vi "teste_command_final.vi"() -> ()   [LabVIEW 2025]
uses:
  <vilib>/Plasmionique/MB Master/MB_Master_Serial/MB_Master_Serial.lvclass
  C:/Program Files/National Instruments/LabVIEW 2025/vi.lib/Plasmionique/MB Master/MB_Master/MB_Master.lvclass
panel:
  out "error out":errorcluster
  in  "habilitar":u16=256
  in  "velocidade":u16
  in  "Serial Config":T1={"baud rate (bps)"=9600, "stop bits"=10, "parity"=2, "flow control"=0, "timeout"=2000, "retries"=3} {"stop bits" items=["1.0"=10, "1.5"=15, "2.0"=20]; "flow control" items=["None", "XON/XOFF", "RTS/CTS", "XON/XOFF & RTS/CTS", "DTR/DSR", "XON/XOFF & DTR/DSR"]; "parity" items=["None", "Odd", "Even", "Mark", "Space"]}
  in  "VISA Resource":refnum<visa-resource-name>="COM3"
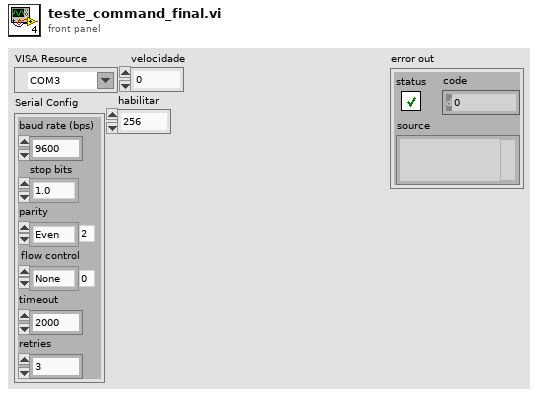
[diagram p1: front panel]
types:
  T1 = cluster{"baud rate (bps)":u32, "stop bits":u16, "parity":u16, "flow control":u16, "timeout":u32, "retries":i32}
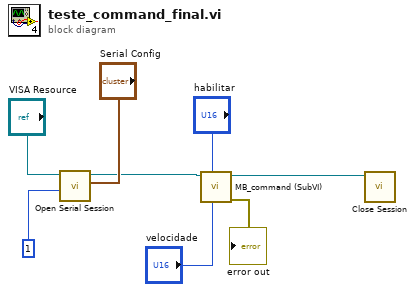
[diagram p0: block diagram]
diagram:
  n1 = call <vilib>:"Open Serial Session.vi"("Slave ID"=u8 1, "Serial Config"="Serial Config", "VISA Resource"="VISA Resource") -> ("MB_Serial session"=w5:refnum<class "MB_Master_Serial.lvclass">)  [unwired: 7 in, 1 out]
  n2 = call "MB_command (SubVI).vi"("velocidade"="velocidade", "habilitar"="habilitar", "MB session in"=w5) -> ("error out"=→"error out":errorcluster, "MB session out"=w2:refnum<class "MB_Master_Serial.lvclass">)  [unwired: 7 in]
  n3 = call-dynamic "Close Session.vi"("MB_Serial session"=w2) -> ()  [unwired: 10 in, 1 out]
